vi "Send Packet.vi"(6 "error in (no error)":errorcluster, 7 "?":T1, 8 "Log string":string, 9 "SerialPortRef":T2) -> (0 "error out":errorcluster, 3 "SerialPortRef out":T2)   [LabVIEW 2016]
uses:
  <vilib>/Rock Robotics/WPI/SerialPort/WPI_SerialPortRef.ctl
  Packet Types.ctl
panel:
  out "Sent string":string
  # "Type:"
  # "Cannot contain line breaks or the character 0x00"
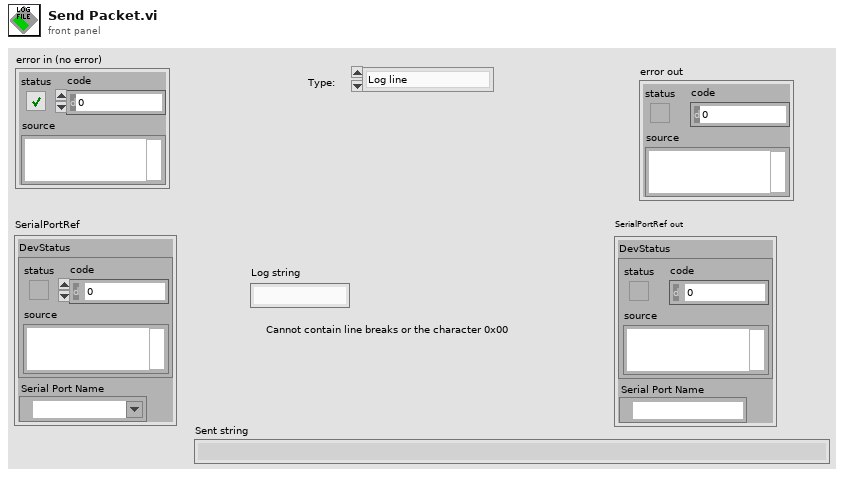
[diagram p1: front panel]
types:
  T1 = typedef "packet types.ctl" = enum16{"Log line", "Open File", "Send Header", "Set Time", "Send to LCD"}
  T2 = typedef "WPI_SerialPortRef.ctl" = cluster{"DevStatus":errorcluster, "Serial Port Name":refnum<visa-resource-name>}
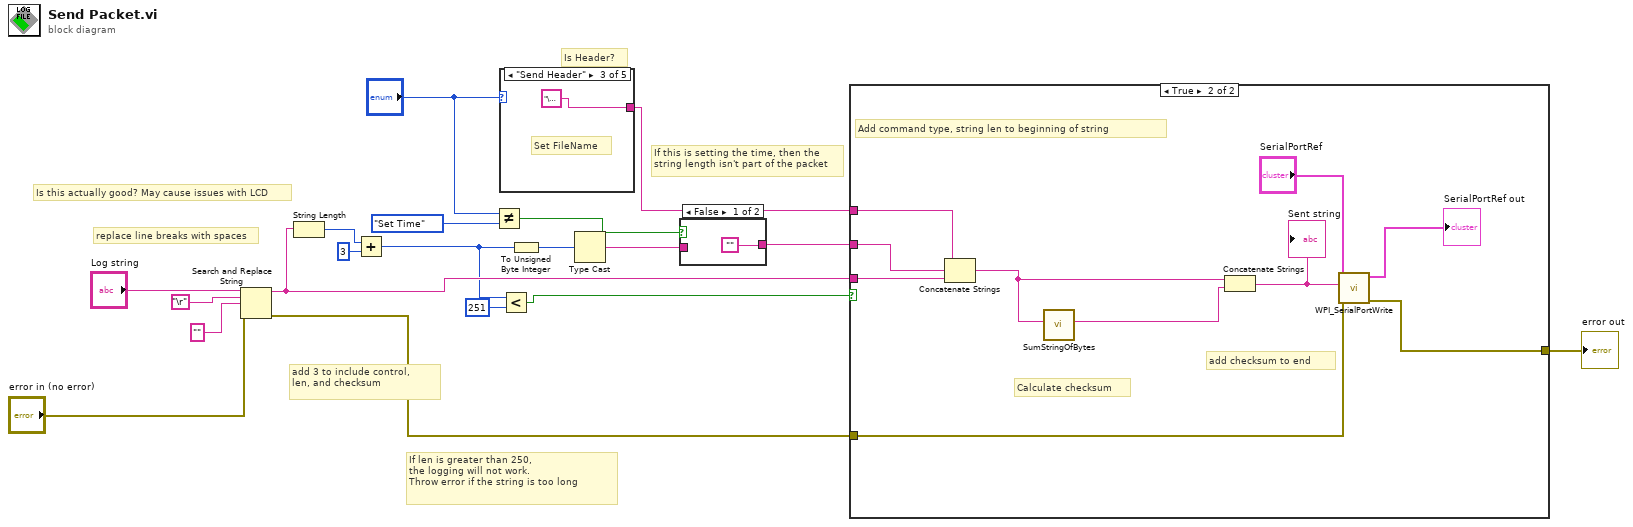
[diagram p0: block diagram]
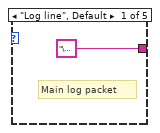
[diagram p3: hidden frame]
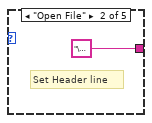
[diagram p4: hidden frame]
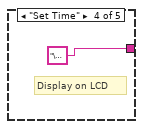
[diagram p5: hidden frame]
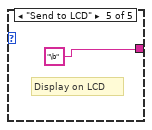
[diagram p6: hidden frame]
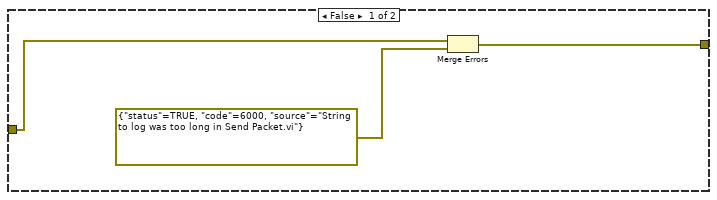
[diagram p7: hidden frame]
diagram:
  # "If this is setting the time, then the \nstring length isn't part of the packet"
  # "Is this actually good? May cause issues with LCD"
  # "Is Header?"
  # "If len is greater than 250,\nthe logging will not work.\nThrow error if the string is too long"
  # "add 3 to include control, \nlen, and checksum"
  # "replace line breaks with spaces"
  n1 = Search and Replace String(input string="Log string", search string="\r", replace string="" ("replace string (\"\")"), error in="error in (no error)") -> (result string=w12:string, error out=w15:errorcluster)  [unwired: 4 in, 2 out]
  n2 = String Length(string=w12) -> (length=w14:i32)
  n3 = Add(x=w14, y=3) -> (x+y=w6:i32)
  n4 = Not Equal?(x="?", y=packet_types."Set Time") -> (x != y?=w1:bool)
  n5 = case shown="\"Send Header\"" "?" {
    tunnel: ["\u0001" ("string") "\u0003" ("string") "\u0002" ("string") "\u0005" ("string") "\b" ("string")] -> w8
    frame "Log line", Default {
      # "Main log packet"
    }
    frame "Open File" {
      # "Set Header line"
    }
    frame "Send Header" {
      # "Set FileName"
    }
    frame "Set Time" {
      # "Display on LCD"
    }
    frame "Send to LCD" {
      # "Display on LCD"
    }
  }
  n6 = Less?(x=w6, y=251) -> (x < y?=w9:bool)
  n7 = To Unsigned Byte Integer(number=w6) -> (unsigned 8bit integer=w7:u8)
  n8 = Type Cast(x=w7) -> (*(type *) &x=w5:string)  [unwired: 1 in]
  n9 = case shown="False" w1 {
    tunnel: w5 -> [_ w26]
    tunnel: ["" w26] -> w4
    frame False {
    }
    frame True {
    }
  }
  n10 = case shown="True" w9 {
    tunnel: w15 -> [w29 w37]
    tunnel: w8 -> [_ w36]
    tunnel: w4 -> [_ w30]
    tunnel: w12 -> [_ w32]
    tunnel: [w27 w31] -> w11
    frame False {
      n11 = Merge Errors(w29, errorcluster {"status"=TRUE, "code"=6000, "source"="String to log was too long in Send Packet.vi"} ("error out")) -> (w27:errorcluster)
    }
    frame True {
      # "add checksum to end"
      # "Add command type, string len to beginning of string"
      # "Calculate checksum"
      n12 = Concatenate Strings(w36, w30, w32) -> (w35:string)
      n13 = call "SumStringOfBytes.vi"("String Of Bytes"=w35) -> ("SumAsString"=w34:string)  [unwired: 10 in]
      n14 = Concatenate Strings(w35, w34) -> (w33:string)
      "Sent string" <- w33
      n15 = call <vilib>:"WPI_SerialPortWrite.vi"("error in (no error)"=w37, "Buffer"=w33, "SerialPortRef"="SerialPortRef") -> ("error out"=w31:errorcluster, "SerialPortRef"=→"SerialPortRef out":T2)  [unwired: 6 in, 1 out]
    }
  }
  "error out" <- w11
